vi "CheckPossibleBalls.vi"(1 "max ball vel":dbl, 7 "timeToValidateBall":dbl=0.5, 9 "Field Size":T3, 10 "Array of cameras":T4[](array[typedef]) {"robots_blue"."height" format="%+4.3f"; "robots_blue"."pixel_y" format="%+4.3f"; "robots_blue"."pixel_x" format="%+4.3f"; "robots_blue"."orientation" format="%+4.3f"; "robots_blue"."y" format="%+4.3f"; "robots_blue"."confidence" format="%4.3f"; "robots_blue"."x" format="%+4.3f"; "robots_yellow"."height" format="%+4.3f"; "robots_yellow"."pixel_y" format="%+4.3f"; "robots_yellow"."pixel_x" format="%+4.3f"; "robots_yellow"."orientation" format="%+4.3f"; "robots_yellow"."y" format="%+4.3f"; "robots_yellow"."confidence" format="%4.3f"; "robots_yellow"."x" format="%+4.3f"}, 11 "last ball choosed by mediacameras":T1[](array[typedef])) -> (2 "sum":i32, 3 "Detection Frame In out":T4[](array[typedef]) {"robots_blue"."height" format="%+4.3f"; "robots_blue"."pixel_y" format="%+4.3f"; "robots_blue"."pixel_x" format="%+4.3f"; "robots_blue"."orientation" format="%+4.3f"; "robots_blue"."y" format="%+4.3f"; "robots_blue"."confidence" format="%4.3f"; "robots_blue"."x" format="%+4.3f"; "robots_yellow"."height" format="%+4.3f"; "robots_yellow"."pixel_y" format="%+4.3f"; "robots_yellow"."pixel_x" format="%+4.3f"; "robots_yellow"."orientation" format="%+4.3f"; "robots_yellow"."y" format="%+4.3f"; "robots_yellow"."confidence" format="%4.3f"; "robots_yellow"."x" format="%+4.3f"})   [LabVIEW 2020]
uses:
  Vision_class/Old vision/Controls/SSL Detection Frame.ctl
  Vision_class/Old vision/Controls/SSL Detection Robot.ctl
  <vilib>/Analysis/Matrix/Datatypes/RealMatrix.ctl
  Vision_class/Old vision/Controls/SSL Detection Ball.ctl
  Utilities_class/Utilities.lvclass
  <vilib>/Analysis/Matrix/NI_Matrix.lvlib
  Vision_class/Vision.lvclass
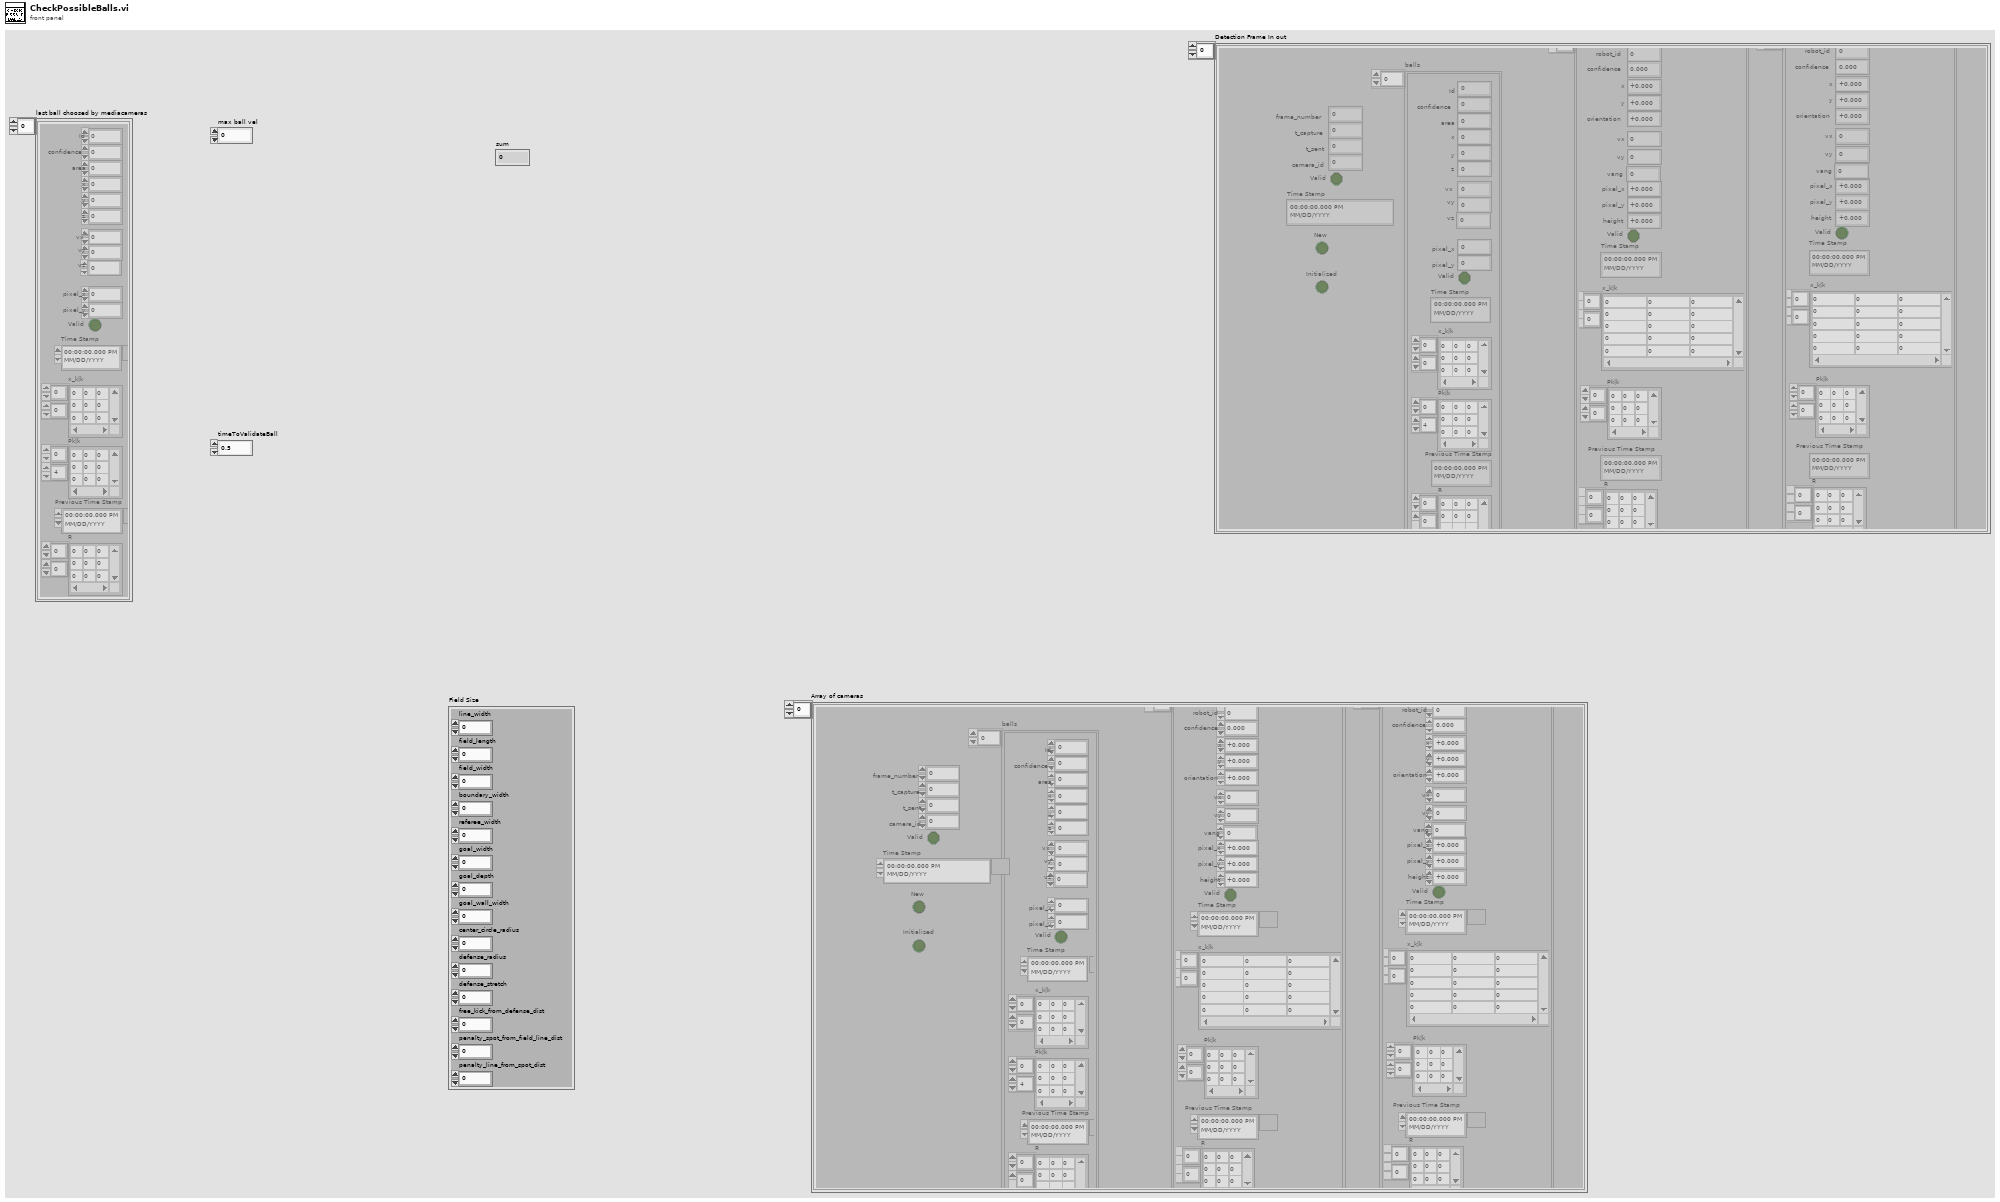
[diagram p1: front panel]
types:
  T1 = typedef "SSL Detection Ball.ctl" = cluster{"x":sgl, "area":u32, "confidence":sgl, "y":sgl, "z":sgl, "pixel_x":sgl, "pixel_y":sgl, "Valid":bool, "Time Stamp":timestamp, "x_k|k":T2, "Pk|k":T2, "Id":u32, "Previous Time Stamp":timestamp, "R":T2, " vx":sgl, "vy":dbl, "vz":dbl}
  T2 = typedef "NI_Matrix.lvlib/RealMatrix.ctl" = dbl[][]
  T3 = cluster{"line_width":u32, "field_length":u32, "field_width":u32, "boundary_width":u32, "referee_width":u32, "goal_width":u32, "goal_depth":u32, "goal_wall_width":u32, "center_circle_radius":u32, "defense_radius":u32, "defense_stretch":u32, "free_kick_from_defense_dist":u32, "penalty_spot_from_field_line_dist":u32, "penalty_line_from_spot_dist":u32}
  T4 = typedef "SSL Detection Frame.ctl" = cluster{"frame_number":u32, "t_capture":dbl, "t_sent":dbl, "camera_id":u32, "robots_yellow":T5[], "robots_blue":T5[], "balls":T1[], "Valid":bool, "Time Stamp":timestamp, "New":bool, "Initialized":bool}
  T5 = typedef "SSL Detection Robot.ctl" = cluster{"x":sgl, "robot_id":u32, "confidence":sgl, "y":sgl, "orientation":sgl, "pixel_x":sgl, "pixel_y":sgl, "height":sgl, "Valid":bool, "Time Stamp":timestamp, "x_k|k":T2, "Pk|k":T2, "Previous Time Stamp":timestamp, "R":T2, "vx":dbl, "vy":dbl, "vang":dbl}
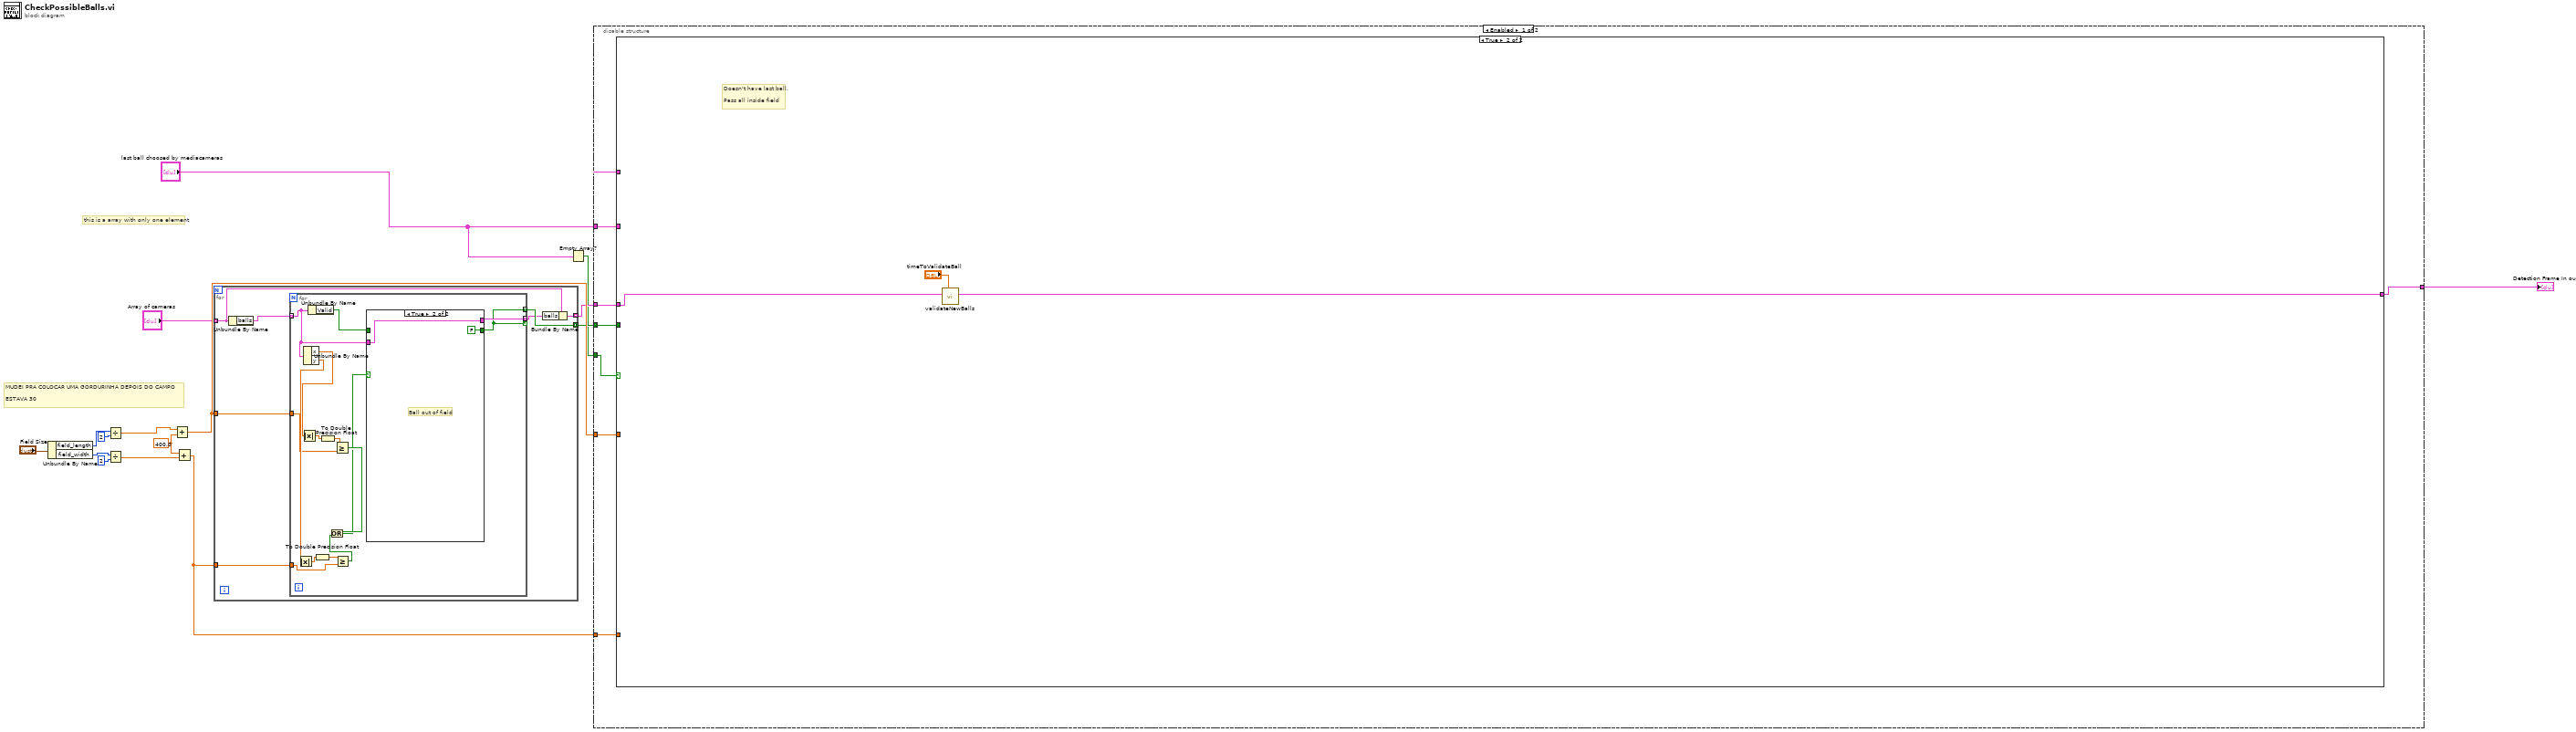
[diagram p0: block diagram]
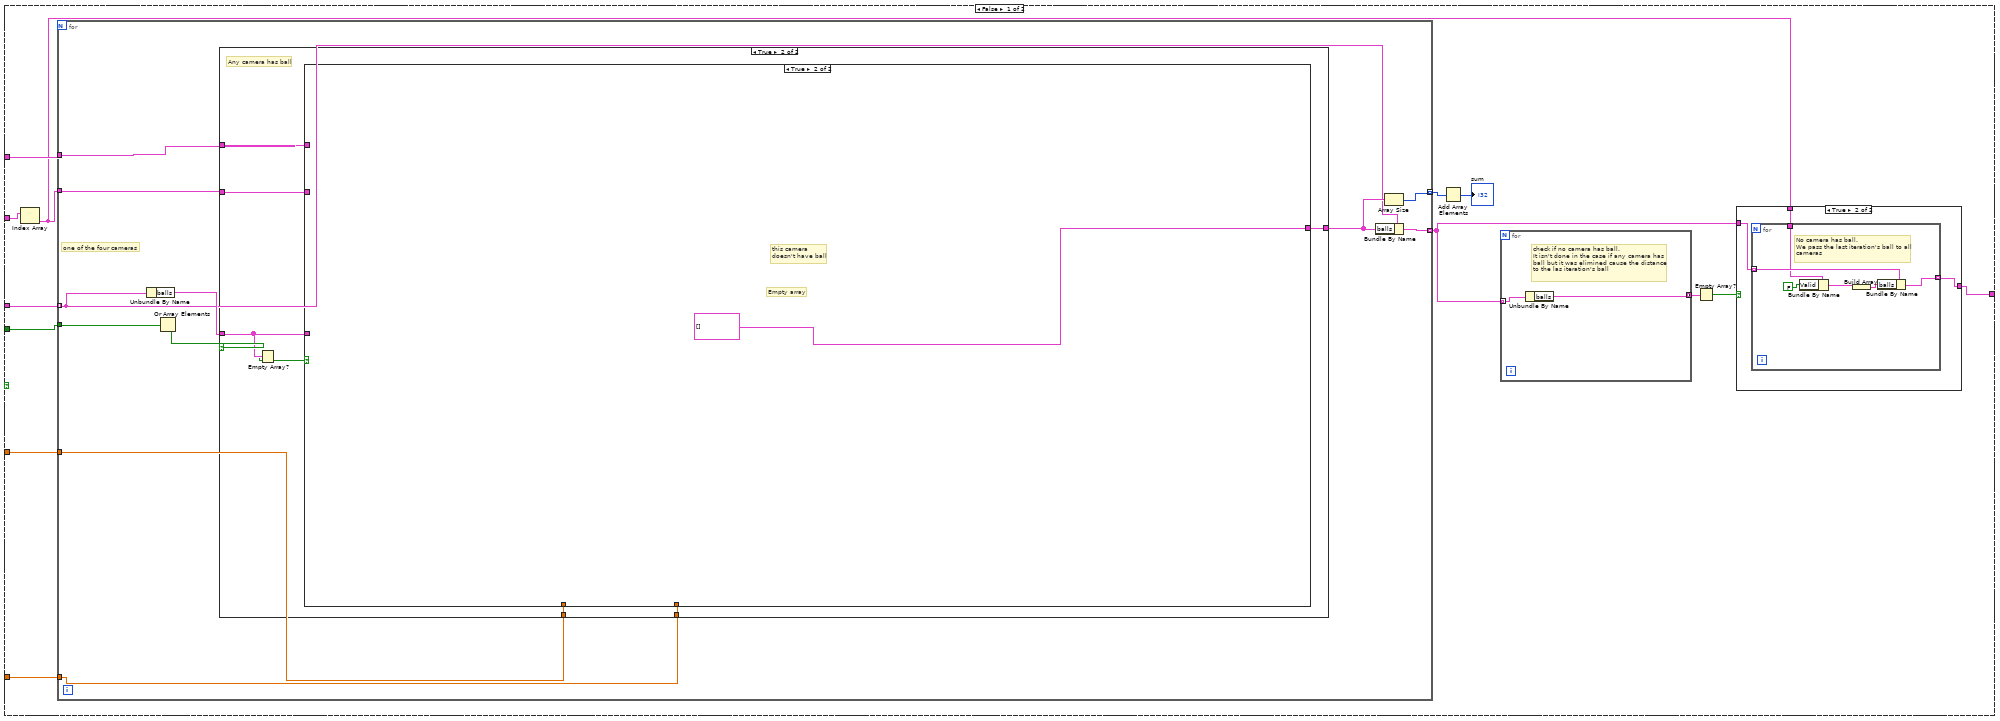
[diagram p2: hidden frame]
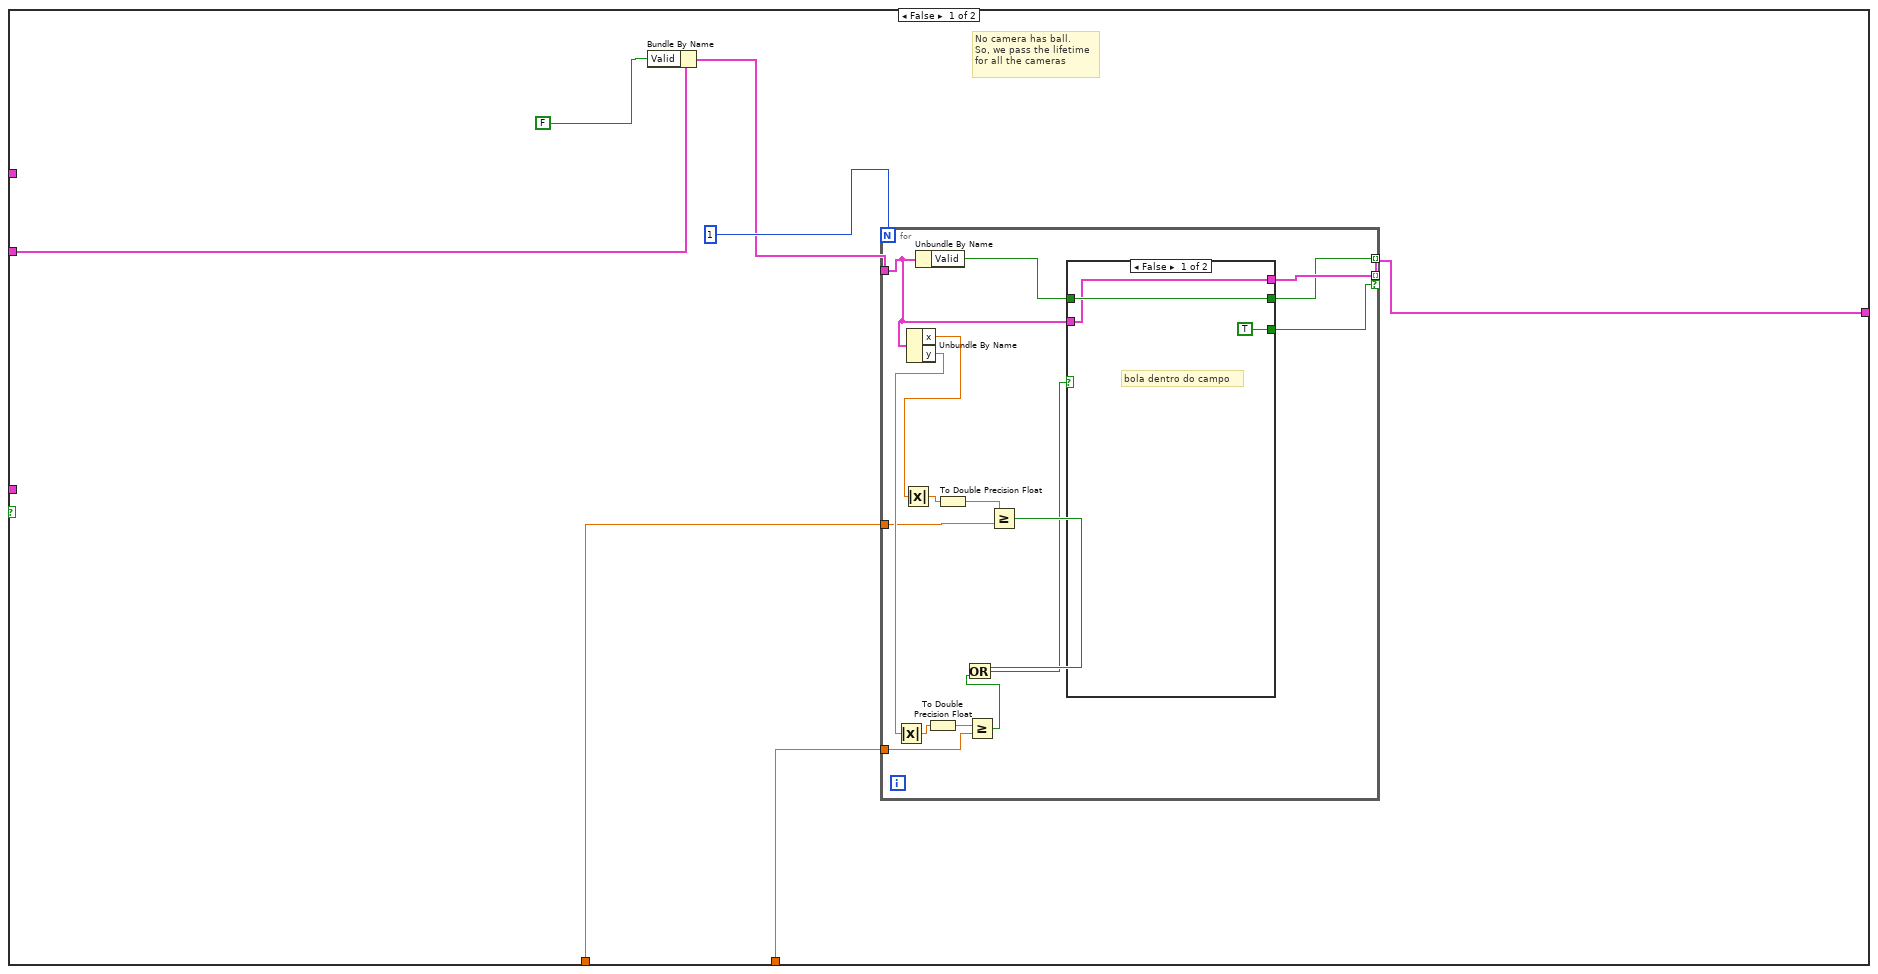
[diagram p3: hidden frame]
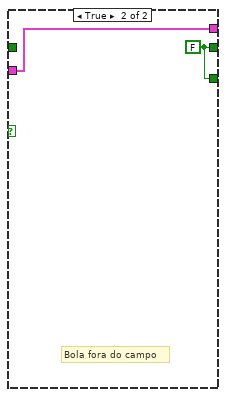
[diagram p4: hidden frame]
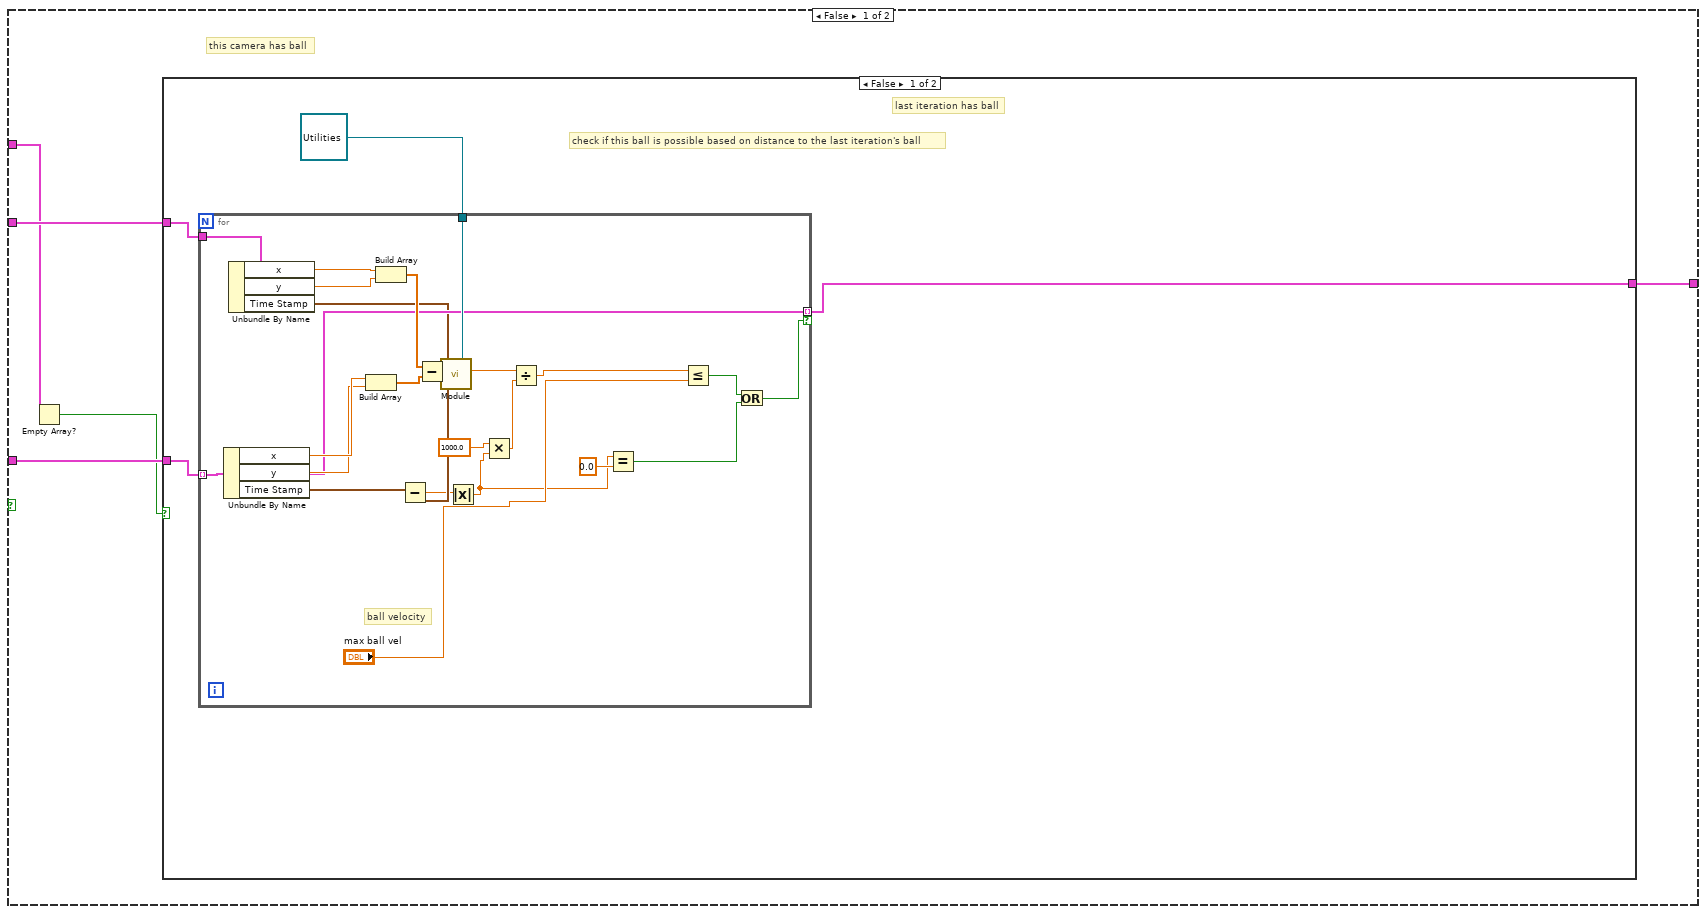
[diagram p5: hidden frame]
diagram:
  w10 = 400.0 ("y")
  # "MUDEI PRA COLOCAR UMA GORDURINHA DEPOIS DO CAMPO\n\nESTAVA 30"
  # "this is a array with only one element"
  n1 = Unbundle By Name("Field Size") -> ("field_length"=w15:u32, "field_width"=w14:u32)
  n2 = Divide(x=w15, y=2) -> (x/y=w1:dbl)
  n3 = Divide(x=w14, y=2) -> (x/y=w11:dbl)
  n4 = Add(x=w1, y=w10) -> (x+y=w8:dbl)
  n5 = Add(x=w10, y=w11) -> (x+y=w9:dbl)
  n6 = for {
    tunnel: w9 -> [w23]
    tunnel: w8 -> [w22]
    tunnel: "Array of cameras" -> [w18] mode=indexing
    tunnel: [w17] -> w5 mode=indexing
    tunnel: [w20] -> w7 mode=concatenating
    n7 = Unbundle By Name(w18) -> ("balls"=w21:T1[])
    n8 = for {
      tunnel: w21 -> [w29] mode=indexing
      tunnel: [w26] -> w20 mode=indexing
      tunnel: [w37] -> w19 mode=indexing if=w26
      tunnel: w23 -> [w25]
      tunnel: w22 -> [w24]
      n9 = Unbundle By Name(w29) -> ("x"=w28:sgl, "y"=w27:sgl)
      n10 = Absolute Value(x=w27) -> (abs(x)=w33:sgl)
      n11 = Absolute Value(x=w28) -> (abs(x)=w32:sgl)
      n12 = Unbundle By Name(w29) -> ("Valid"=w38:bool)
      n13 = To Double Precision Float(number=w33) -> (double precision float=w34:dbl)
      n14 = To Double Precision Float(number=w32) -> (double precision float=w31:dbl)
      n15 = Greater Or Equal?(x=w31, y=w24) -> (x >= y?=w36:bool)
      n16 = Greater Or Equal?(x=w34, y=w25) -> (x >= y?=w35:bool)
      n17 = Or(x=w36, y=w35) -> (x .or. y?=w30:bool)
      n18 = case shown="True" w30 {
        tunnel: w38 -> [w40 _]
        tunnel: [w40 FALSE ("Valid")] -> w26
        tunnel: w29 -> [w39 w41]
        tunnel: [w39 w41] -> w37
        frame False {
          # "ball inside field"
        }
        frame True {
          # "Ball out of field"
        }
      }
    }
    n19 = Bundle By Name(cluster=w18, "balls"=w19) -> (w17:T4)
  }
  n20 = Empty Array?(array="last ball choosed by mediacameras") -> (empty?=w4:bool)
  n21 = disable-structure shown="Enabled" {
    disable-tunnel: w9 -> [w49 _]
    disable-tunnel: w8 -> [w48 _]
    disable-tunnel: w7 -> [w47 _]
    disable-tunnel: w5 -> [w46 w158]
    disable-tunnel: w4 -> [w45 _]
    disable-tunnel: "last ball choosed by mediacameras" -> [w44 _]
    disable-tunnel: [w43 w158] -> w2
    frame Enabled {
      n22 = case shown="True" w45 {
        tunnel: w49 -> [w60 _]
        tunnel: w48 -> [w59 _]
        tunnel: w47 -> [w58 _]
        tunnel: w44 -> [w54 _]
        tunnel: [w50 w156] -> w43
        tunnel: w46 -> [w53 w157]
        tunnel: w44 -> [w52 _]
        frame False {
          n23 = Index Array(array=w52) -> (element=w51:T1)  [unwired: 1 in]
          n24 = for {
            tunnel: [w72] -> w55 mode=indexing
            tunnel: w54 -> [w71]
            tunnel: [w69] -> w62 mode=indexing
            tunnel: w60 -> [w68]
            tunnel: w59 -> [w67]
            tunnel: w58 -> [w65]
            tunnel: w53 -> [w64] mode=indexing
            tunnel: w51 -> [w63]
            # "one of the four cameras"
            n25 = Unbundle By Name(w64) -> ("balls"=w66:T1[])
            n26 = Or Array Elements(Boolean array=w65) -> (logical OR=w73:bool)
            n27 = case shown="True" w73 {
              tunnel: w66 -> [_ w103]
              tunnel: w63 -> [w80 w108]
              tunnel: w71 -> [_ w106]
              tunnel: [w74 w107] -> w70
              tunnel: w67 -> [w76 w105]
              tunnel: w68 -> [w75 w104]
              frame False {
                # "No camera has ball.\nSo, we pass the lifetime\nfor all the cameras"
                n28 = Bundle By Name(cluster=w80, "Valid"=FALSE) -> (w77:T1)
                n29 = for {
                  N: 1 -> [_]
                  tunnel: w77 -> [w87]
                  tunnel: [w82] -> _ mode=indexing
                  tunnel: [w95] -> w74 mode=indexing if=w81
                  tunnel: w76 -> [w84]
                  tunnel: w75 -> [w83]
                  n30 = Unbundle By Name(w87) -> ("x"=w86:sgl, "y"=w85:sgl)
                  n31 = Absolute Value(x=w85) -> (abs(x)=w91:sgl)
                  n32 = Absolute Value(x=w86) -> (abs(x)=w90:sgl)
                  n33 = Unbundle By Name(w87) -> ("Valid"=w96:bool)
                  n34 = To Double Precision Float(number=w91) -> (double precision float=w92:dbl)
                  n35 = To Double Precision Float(number=w90) -> (double precision float=w89:dbl)
                  n36 = Greater Or Equal?(x=w92, y=w83) -> (x >= y?=w93:bool)
                  n37 = Greater Or Equal?(x=w89, y=w84) -> (x >= y?=w94:bool)
                  n38 = Or(x=w94, y=w93) -> (x .or. y?=w88:bool)
                  n39 = case shown="False" w88 {
                    tunnel: w96 -> [w99 _]
                    tunnel: [w99 w100] -> w82
                    tunnel: w87 -> [w98 w101]
                    tunnel: [w98 w101] -> w95
                    tunnel: [TRUE w100] -> w81
                    frame False {
                      # "bola dentro do campo"
                    }
                    frame True {
                      w100 = FALSE ("Valid")
                      # "Bola fora do campo"
                    }
                  }
                }
              }
              frame True {
                # "Any camera has ball"
                n40 = Empty Array?(array=w103) -> (empty?=w102:bool)
                n41 = case shown="True" w102 {
                  tunnel: w103 -> [w113 _]
                  tunnel: w108 -> [w112 _]
                  tunnel: [w111 T1[] [] ("balls")] -> w107
                  tunnel: w106 -> [w110 _]
                  tunnel: w105 -> [_ _]
                  tunnel: w104 -> [_ _]
                  frame False {
                    # "this camera has ball"
                    n42 = Empty Array?(array=w110) -> (empty?=w109:bool)
                    n43 = case shown="False" w109 {
                      tunnel: w113 -> [w117 w141]
                      tunnel: w112 -> [w116 _]
                      tunnel: [w114 w141] -> w111
                      frame False {
                        # "check if this ball is possible based on distance to the last iteration's ball"
                        # "last iteration has ball"
                        n44 = for {
                          tunnel: w117 -> [w131] mode=indexing
                          tunnel: w116 -> [w140]
                          tunnel: refnum<class "Utilities.lvclass"> refnum ("Utilities in") -> [w133]
                          tunnel: [w131] -> w114 mode=indexing if=w122
                          # "ball velocity"
                          n45 = Unbundle By Name(w131) -> ("x"=w139:sgl, "y"=w138:sgl, "Time Stamp"=w130:timestamp)
                          n46 = Unbundle By Name(w140) -> ("x"=w137:sgl, "y"=w136:sgl, "Time Stamp"=w129:timestamp)
                          n47 = Build Array(w139, w138) -> (w134:sgl[])
                          n48 = Build Array(w137, w136) -> (w135:sgl[])
                          n49 = Subtract(x=w129, y=w130) -> (x-y=w128:dbl)
                          n50 = Subtract(x=w135, y=w134) -> (x-y=w132:sgl[])
                          n51 = call "Module.vi"("2D vector"=w132, "Utilities in"=w133) -> ("Modulo"=w127:dbl)  [unwired: 7 in, 2 out]
                          n52 = Absolute Value(x=w128) -> (abs(x)=w118:dbl)
                          n53 = Multiply(x=1000.0, y=w118) -> (x*y=w126:dbl)
                          n54 = Divide(x=w127, y=w126) -> (x/y=w119:dbl)
                          n55 = Equal?(x=w118, y=0.0) -> (x = y?=w124:bool)
                          n56 = Less Or Equal?(x=w119, y="max ball vel") -> (x <= y?=w123:bool)
                          n57 = Or(x=w123, y=w124) -> (x .or. y?=w122:bool)
                        }
                      }
                      frame True {
                        # "last iteration doesn't have ball,\nincluding the first iteration.\n\nSo, we pass all balls. If it's in this case, that's why this camera has ball."
                      }
                    }
                  }
                  frame True {
                    # "Empty array"
                    # "this camera \ndoesn't have ball"
                  }
                }
              }
            }
            n58 = Bundle By Name(cluster=w64, "balls"=w70) -> (w72:T4)
            n59 = Array Size(array=w70) -> (size(s)=w69:i32)
          }
          n60 = Add Array Elements(numeric array=w62) -> (sum=→"sum":i32)
          n61 = for {
            tunnel: w55 -> [w154] mode=indexing
            tunnel: [w153] -> w57 mode=concatenating
            # "check if no camera has ball.\nIt isn't done in the case if any camera has\nball but it was elimined cause the distance\nto the las iteration's ball"
            n62 = Unbundle By Name(w154) -> ("balls"=w153:T1[])
          }
          n63 = Empty Array?(array=w57) -> (empty?=w56:bool)
          n64 = case shown="True" w56 {
            tunnel: [w143 w145] -> w50
            tunnel: w55 -> [w143 w146]
            tunnel: w51 -> [_ w144]
            frame False {
              # "any camera has ball"
            }
            frame True {
              n65 = for {
                tunnel: w146 -> [w152] mode=indexing
                tunnel: [w151] -> w145 mode=indexing
                tunnel: w144 -> [w149]
                # "No camera has ball.\nWe pass the last iteration's ball to all\ncameras"
                n66 = Bundle By Name(cluster=w149, "Valid"=FALSE) -> (w148:T1)
                n67 = Build Array(w148) -> (w150:T1[])
                n68 = Bundle By Name(cluster=w152, "balls"=w150) -> (w151:T4)
              }
            }
          }
        }
        frame True {
          # "Doesn't have last ball.\n\nPass all inside field"
          n69 = call "validateNewBalls.vi"("timeToValidateBall"="timeToValidateBall", "array of cameras in"=w157) -> ("Array of cameras out"=w156:T4[])  [unwired: 7 in, 2 out]
        }
      }
    }
    frame Disabled {
    }
  }
  "Detection Frame In out" <- w2
